vi "AutoApproach.vi"() -> ()   [LabVIEW 2019]
doc: "Programming Interface Example: Automatic approach implemented using Nanonis Programming Interface functions. This can be used if you want to execute special functions after each motor step or if you want to control your motor directly from LabVIEW.\n\n- Nanonis Programming Interface -"
uses:
  GlobalClicksHeight.vi
  <userlib>/Nanonis Prog Interface V5/Nanonis Prog Interface.lvlib
panel:
  in  "stop":bool
  out "Surface reached":bool
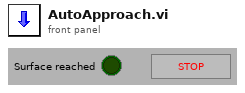
[diagram p1: front panel]
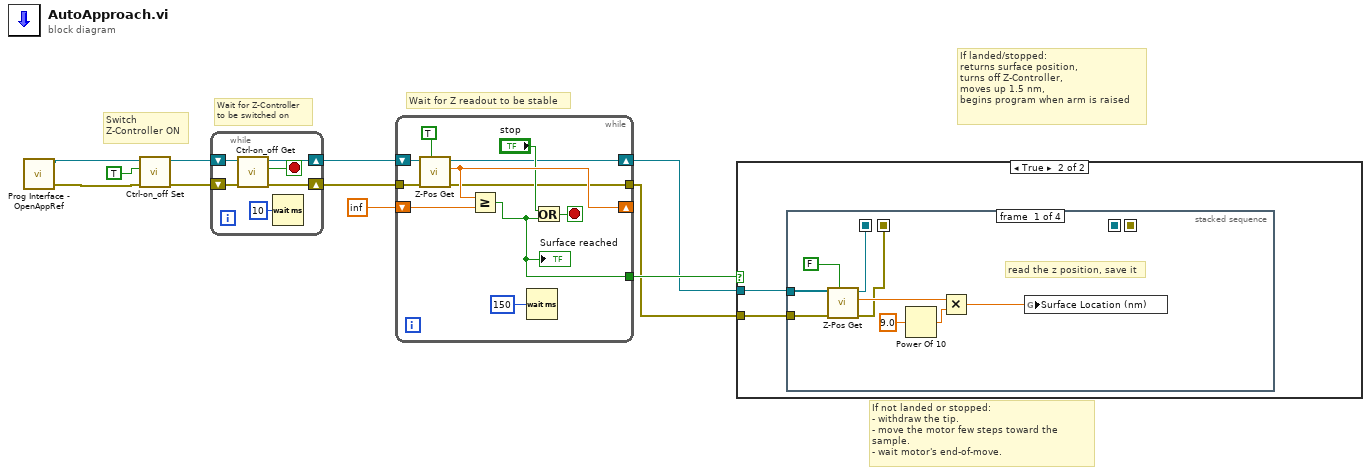
[diagram p0: block diagram]
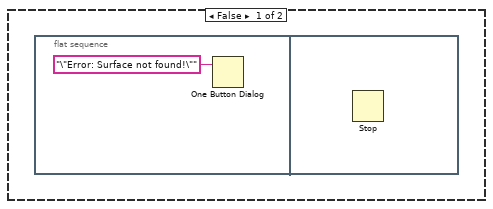
[diagram p2: hidden frame]
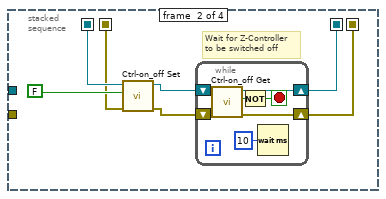
[diagram p3: hidden frame]
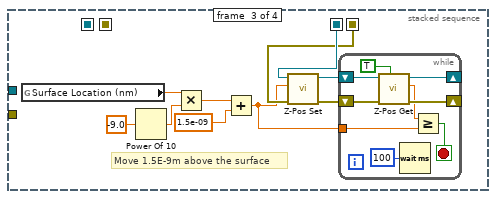
[diagram p4: hidden frame]
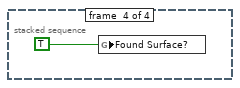
[diagram p5: hidden frame]
diagram:
  # "Wait for Z readout to be stable"
  # "If landed/stopped:  \nreturns surface position, \nturns off Z-Controller, \nmoves up 1.5 nm,\nbegins program when arm is raised"
  # "Wait for Z-Controller\nto be switched on"
  # "Switch Z-Controller ON"
  # "If not landed or stopped:\n- withdraw the tip.\n- move the motor few steps toward the sample.\n- wait motor's end-of-move."
  n1 = call <userlib>:"Prog Interface - OpenAppRef.vi"() -> ("Error out"=w10:errorcluster, "Application reference"=w11:refnum<vi>)  [unwired: 6 in]
  n2 = call <userlib>:"Ctrl-on_off Set.vi"("error in (no error)"=w10, "Z Controller ON/OFF"=TRUE ("Ctrl on/off"), "Application ref in"=w11) -> ("error out"=w6:errorcluster, "Application ref out"=w4:refnum<vi>)  [unwired: 7 in]
  n3 = while {
    shift-right: [w17] -> w5
    shift-left: w6 -> [w16]
    shift-right: [w12] -> w3
    shift-left: w4 -> [w13]
    stop <- w15 stop-if-true
    n4 = call <userlib>:"Ctrl-on_off Get.vi"("error in (no error)"=w16, "Application ref in"=w13) -> ("error out"=w17:errorcluster, "Z-Controller on/off status"=w15:bool, "Application ref out"=w12:refnum<vi>)  [unwired: 7 in]
    n5 = Wait (ms)(milliseconds to wait=u32 10) -> ()  [unwired: 1 out]
  }
  n6 = while {
    shift-right: [w26] -> _
    shift-left: sgl inf ("Z-pos (m)") -> [w28]
    tunnel: [w20] -> w9
    tunnel: w5 -> [w24]
    shift-right: [w22] -> w2
    shift-left: w3 -> [w23]
    tunnel: [w19] -> w1
    stop <- w21 stop-if-true
    n7 = call <userlib>:"Z-Pos Get.vi"("Wait for newest data (F=False)"=TRUE, "error in (no error)"=w24, "Application ref in"=w23) -> ("error out"=w19:errorcluster, "Z position (m)"=w26:sgl, "Application ref out"=w22:refnum<vi>)  [unwired: 6 in]
    n8 = Greater Or Equal?(x=w26, y=w28) -> (x >= y?=w20:bool)
    "Surface reached" <- w20
    n9 = Wait (ms)(milliseconds to wait=u32 150) -> ()  [unwired: 1 out]
    n10 = Or(x="stop", y=w20) -> (x .or. y?=w21:bool)
  }
  n11 = case shown="True" w9 {
    tunnel: w2 -> [_ w31]
    tunnel: w1 -> [_ w30]
    frame False {
      n12 = flat-sequence {
        frame #0 {
          n13 = One Button Dialog(message="\"Error: Surface not found!\"") -> ()  [unwired: 1 in, 1 out]
        }
        frame #1 {
          n14 = Stop() -> ()  [unwired: 1 in]
        }
      }
    }
    frame True {
      n15 = stacked-sequence {
        seq-local: [w37 _ _ _] -> [_ w46 _ _]
        seq-local: [w35 _ _ _] -> [_ w45 _ _]
        seq-local: [_ w42 _ _] -> [_ _ w60 _]
        seq-local: [_ w41 _ _] -> [_ _ w59 _]
        tunnel: w31 -> [w36 _ _ _]
        tunnel: w30 -> [w33 _ _ _]
        frame #0 {
          # "read the z position, save it"
          n16 = call <userlib>:"Z-Pos Get.vi"("Wait for newest data (F=False)"=FALSE, "error in (no error)"=w33, "Application ref in"=w36) -> ("error out"=w35:errorcluster, "Z position (m)"=w40:sgl, "Application ref out"=w37:refnum<vi>)  [unwired: 6 in]
          n17 = Power Of 10(x=9.0) -> (10^x=w39:dbl)
          n18 = Multiply(x=w40, y=w39) -> (x*y=w34:dbl)
          n19 = global write "GlobalClicksHeight.vi" "Surface Location (nm)"(w34) -> ()
        }
        frame #1 {
          # "Wait for Z-Controller\nto be switched off"
          n20 = call <userlib>:"Ctrl-on_off Set.vi"("error in (no error)"=w45, "Z Controller ON/OFF"=FALSE, "Application ref in"=w46) -> ("error out"=w43:errorcluster, "Application ref out"=w44:refnum<vi>)  [unwired: 7 in]
          n21 = while {
            shift-right: [w54] -> w41
            shift-left: w43 -> [w53]
            shift-right: [w49] -> w42
            shift-left: w44 -> [w50]
            stop <- w48 stop-if-true
            n22 = call <userlib>:"Ctrl-on_off Get.vi"("error in (no error)"=w53, "Application ref in"=w50) -> ("error out"=w54:errorcluster, "Z-Controller on/off status"=w52:bool, "Application ref out"=w49:refnum<vi>)  [unwired: 7 in]
            n23 = Not(x=w52) -> (.not. x?=w48:bool)
            n24 = Wait (ms)(milliseconds to wait=u32 10) -> ()  [unwired: 1 out]
          }
        }
        frame #2 {
          # "Move 1.5E-9m above the surface"
          n25 = global read "GlobalClicksHeight.vi" "Surface Location (nm)"() -> (w55:dbl)
          n26 = Power Of 10(x=-9.0) -> (10^x=w64:dbl)
          n27 = Multiply(x=w55, y=w64) -> (x*y=w62:dbl)
          n28 = Add(x=w62, y=1.5e-09) -> (x+y=w56:dbl)
          n29 = call <userlib>:"Z-Pos Set.vi"("error in (no error)"=w59, "Z position (m)"=w56, "Application ref in"=w60) -> ("error out"=w57:errorcluster, "Application ref out"=w58:refnum<vi>)  [unwired: 7 in]
          n30 = while {
            shift-right: [w70] -> _
            shift-left: w57 -> [w72]
            shift-right: [w71] -> _
            shift-left: w58 -> [w73]
            tunnel: w56 -> [w67]
            stop <- w69 stop-if-true
            n31 = call <userlib>:"Z-Pos Get.vi"("Wait for newest data (F=False)"=TRUE, "error in (no error)"=w72, "Application ref in"=w73) -> ("error out"=w70:errorcluster, "Z position (m)"=w68:sgl, "Application ref out"=w71:refnum<vi>)  [unwired: 6 in]
            n32 = Wait (ms)(milliseconds to wait=u32 100) -> ()  [unwired: 1 out]
            n33 = Greater Or Equal?(x=w68, y=w67) -> (x >= y?=w69:bool)
          }
        }
        frame #3 {
          n34 = global write "GlobalClicksHeight.vi" "Found Surface?"(TRUE ("Clicks and Height")) -> ()
        }
      }
    }
  }
